vi "prova acq 2.vi"() -> ()   [LabVIEW 2019]
uses:
  <vilib>/DAQmx/read.llb/DAQmx Read (Analog 1D Wfm NChan NSamp).vi
  <vilib>/DAQmx/create/channels.llb/DAQmx Create Channel (AI-Voltage-Basic).vi
  <vilib>/DAQmx/configure/timing.llb/DAQmx Timing (Sample Clock).vi
  <vilib>/DAQmx/miscellaneous.llb/DAQmx Fill In Error Info.vi
panel:
  in  "samples per channel":i32=500000
  out "Numeric":i32
  out "Array":i32[](array[numeric])
  in  "error in":errorcluster
  in  "MODULE NAME":string="cDAQ9181-1B4068CMod1"
  in  "stop":bool
  in  "millisecond multiple":u32
  out "Waveform Chart":waveform(dbl)[](graph)
  in  "sample mode":i32(ring)=10123 items=["Finite Samples"=10178, "Continuous Samples"=10123, "Hardware Timed Single Point"=12522]
  in  "rate":dbl=20000.0 format="%0.2f"
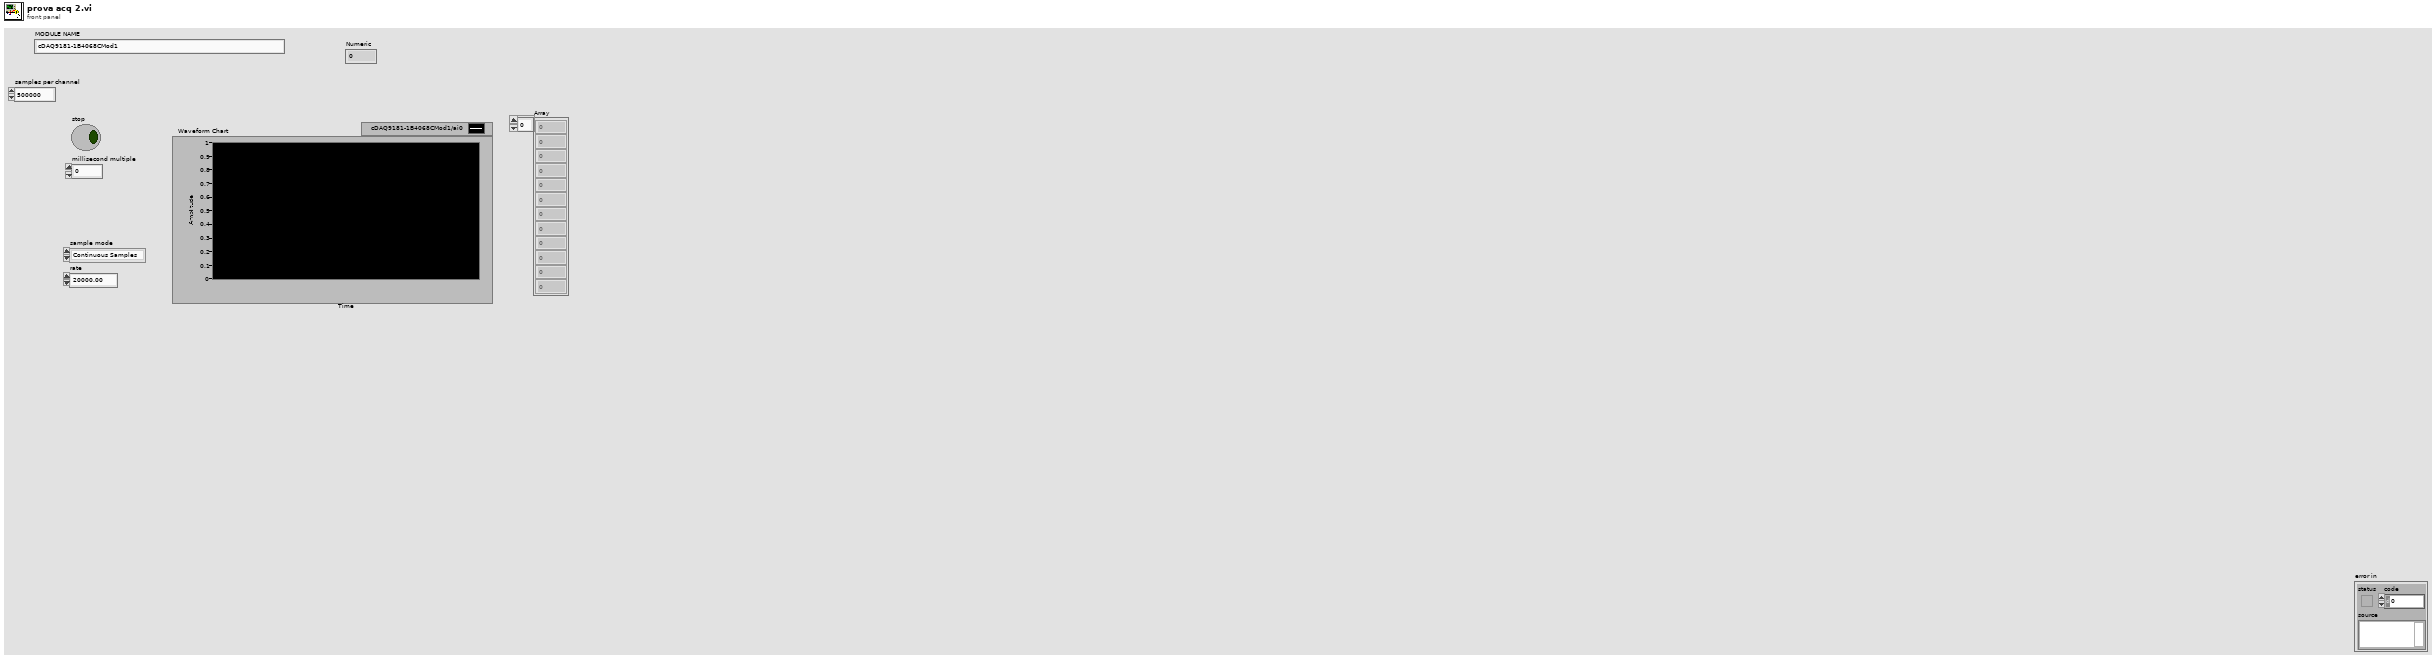
[diagram p1: front panel]
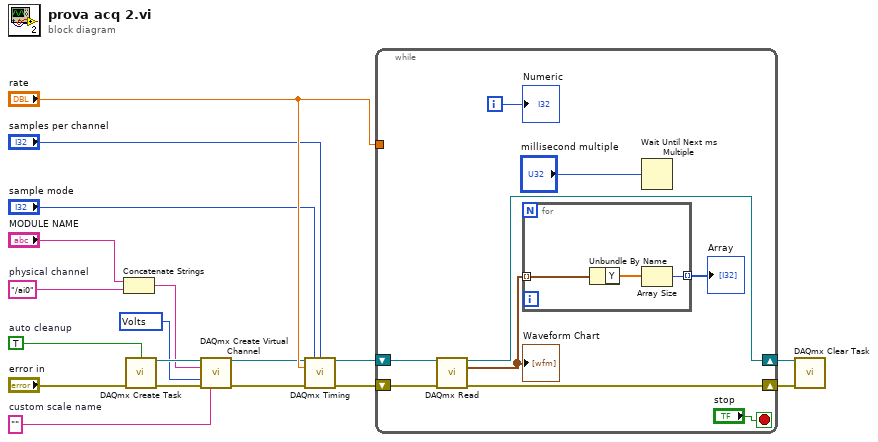
[diagram p0: block diagram]
diagram:
  w4 = 10348 items=["Volts"=10348, "From Custom Scale"=10065] ("units")
  w7 = ""  # custom scale name
  w6 = "/ai0"  # physical channel
  w9 = TRUE  # auto cleanup
  n1 = Concatenate Strings("MODULE NAME", w6) -> (w5:string)
  n2 = call <vilib>:"DAQmx Create Task.vi"("auto cleanup"=w9, "error in"="error in") -> ("task out"=w8:refnum<k21>, "error out"=w10:errorcluster)  [unwired: 12 in]
  n3 = call-poly <vilib>:"DAQmx Create Virtual Channel.vi"("task in"=w8, "physical channels"=w5, "units"=w4, "error in"=w10, "custom scale name"=w7) -> ("task out"=w13:refnum<k21>, "error out"=w14:errorcluster)  [unwired: 9 in]
  n4 = call-poly <vilib>:"DAQmx Timing.vi"("task/channels in"=w13, "sample mode"="sample mode", "samples per channel"="samples per channel", "rate"="rate", "error in"=w14) -> ("task out"=w15:refnum<k21>, "error out"=w16:errorcluster)  [unwired: 9 in]
  n5 = while {
    shift-right: [w27] -> w3
    shift-left: w15 -> [w20]
    shift-right: [w25] -> w2
    shift-left: w16 -> [w26]
    tunnel: "rate" -> [_]
    i -> [w21]
    stop <- "stop" stop-if-true
    n6 = call-poly <vilib>:"DAQmx Read.vi"("task/channels in"=w20, "error in"=w26) -> ("task out"=w27:refnum<k21>, "data"=w23:waveform(dbl)[], "error out"=w25:errorcluster)  [unwired: 11 in]
    "Waveform Chart" <- w23
    n7 = for {
      tunnel: w23 -> [w30] mode=indexing
      tunnel: [w28] -> w22 mode=indexing
      n8 = Unbundle By Name(w30) -> ("Y"=w29:dbl[])
      n9 = Array Size(array=w29) -> (size(s)=w28:i32)
    }
    "Array" <- w22
    n10 = Wait Until Next ms Multiple(millisecond multiple="millisecond multiple") -> ()  [unwired: 1 out]
    "Numeric" <- w21
  }
  n11 = call <vilib>:"DAQmx Clear Task.vi"("task in"=w3, "error in"=w2) -> ()  [unwired: 13 in, 1 out]
